vi "Initialize RF Sessions.vi"(0 "RF Subsystem Session Provider in":refnum<class "RF Subsystem Session Provider.lvclass">, 5 "TSM Context":T1, 11 "error in":errorcluster) -> (4 "RF Subsystem Session Provider out":refnum<class "RF Subsystem Session Provider.lvclass">, 15 "error out":errorcluster)   [LabVIEW 2023, in "RFFixtureCharact.RFPM.lvlib" / "RF Subsystem Session Provider.lvclass"]
uses:
  RF Subsystem Session Provider.lvclass
  <vilib>/NI_TestStand_SemiconductorModule/NI_TestStand_Semiconductor_Module.lvlibp/PinMap/General/SemiconductorModuleContext.ctl
  Controls/RFPM Settings.ctl
  Controls/Calibration Check.ctl
  Common/RF Subsystem Session Provider/Utilities/Global Data Id Prefix.vi
  <vilib>/NI_TestStand_SemiconductorModule/NI_TestStand_Semiconductor_Module.lvlibp/PinMap/Site and Global Data/SetGlobalData.vi
  RF Subsystem Session Provider.lvclass/RF Subsystem Session Provider.ctl
  Common/RFCalAndFixtureCharact.Common.lvlib
  <vilib>/NI_TestStand_SemiconductorModule/NI_TestStand_Semiconductor_Module.lvlibp
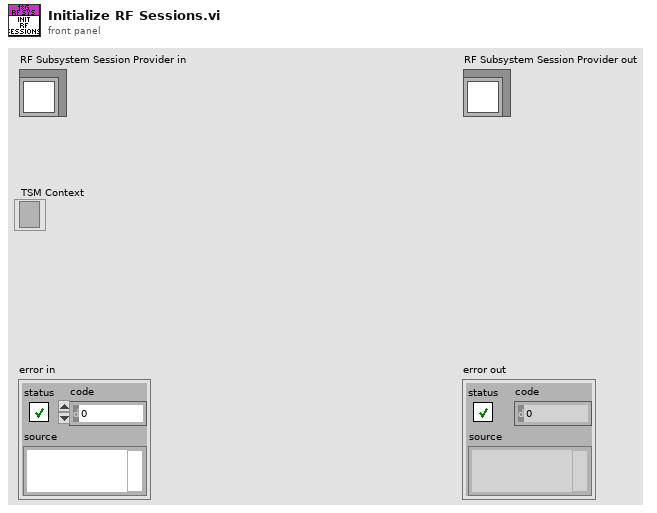
[diagram p1: front panel]
types:
  T1 = typedef "NI_TestStand_Semiconductor_Module.lvlibp/SemiconductorModuleContext.ctl" = refnum<k7>
  T2 = enum16{"OnboardClock", "RefIn", "PXI_Clk", "ClkIn", "RefIn2", "PXI_ClkMaster"}
  T3 = typedef "RFFixtureCharact.RFPM.lvlib/RF Subsystem Session Provider.lvclass/RFPM Settings.ctl" = cluster{"Suppress System Calibration?":bool, "User-Defined Calibration":cluster{"Frequency Interpolation Enabled":bool, "Maximum Frequency Span for Interpolation":dbl, "Source Power Level Coercion Method":i32, "Maximum Source Power Level Coercion":dbl, "Receiver Reference Level Coercion Enabled":bool, "Maximum Receiver Reference Level Coercion":dbl, "Calibration File VST Serial Must Match":bool, "Calibration Interval Check":T4}}
  T4 = typedef "RFFixtureCharact.RFPM.lvlib/RF Subsystem Session Provider.lvclass/Calibration Check.ctl" = cluster{"Check Calibration Interval?":bool, "Temperature Interval (deg C)":dbl, "Calibration Interval (days)":dbl, "Out of Calibration Message":enum16{"Warning", "Error"}}
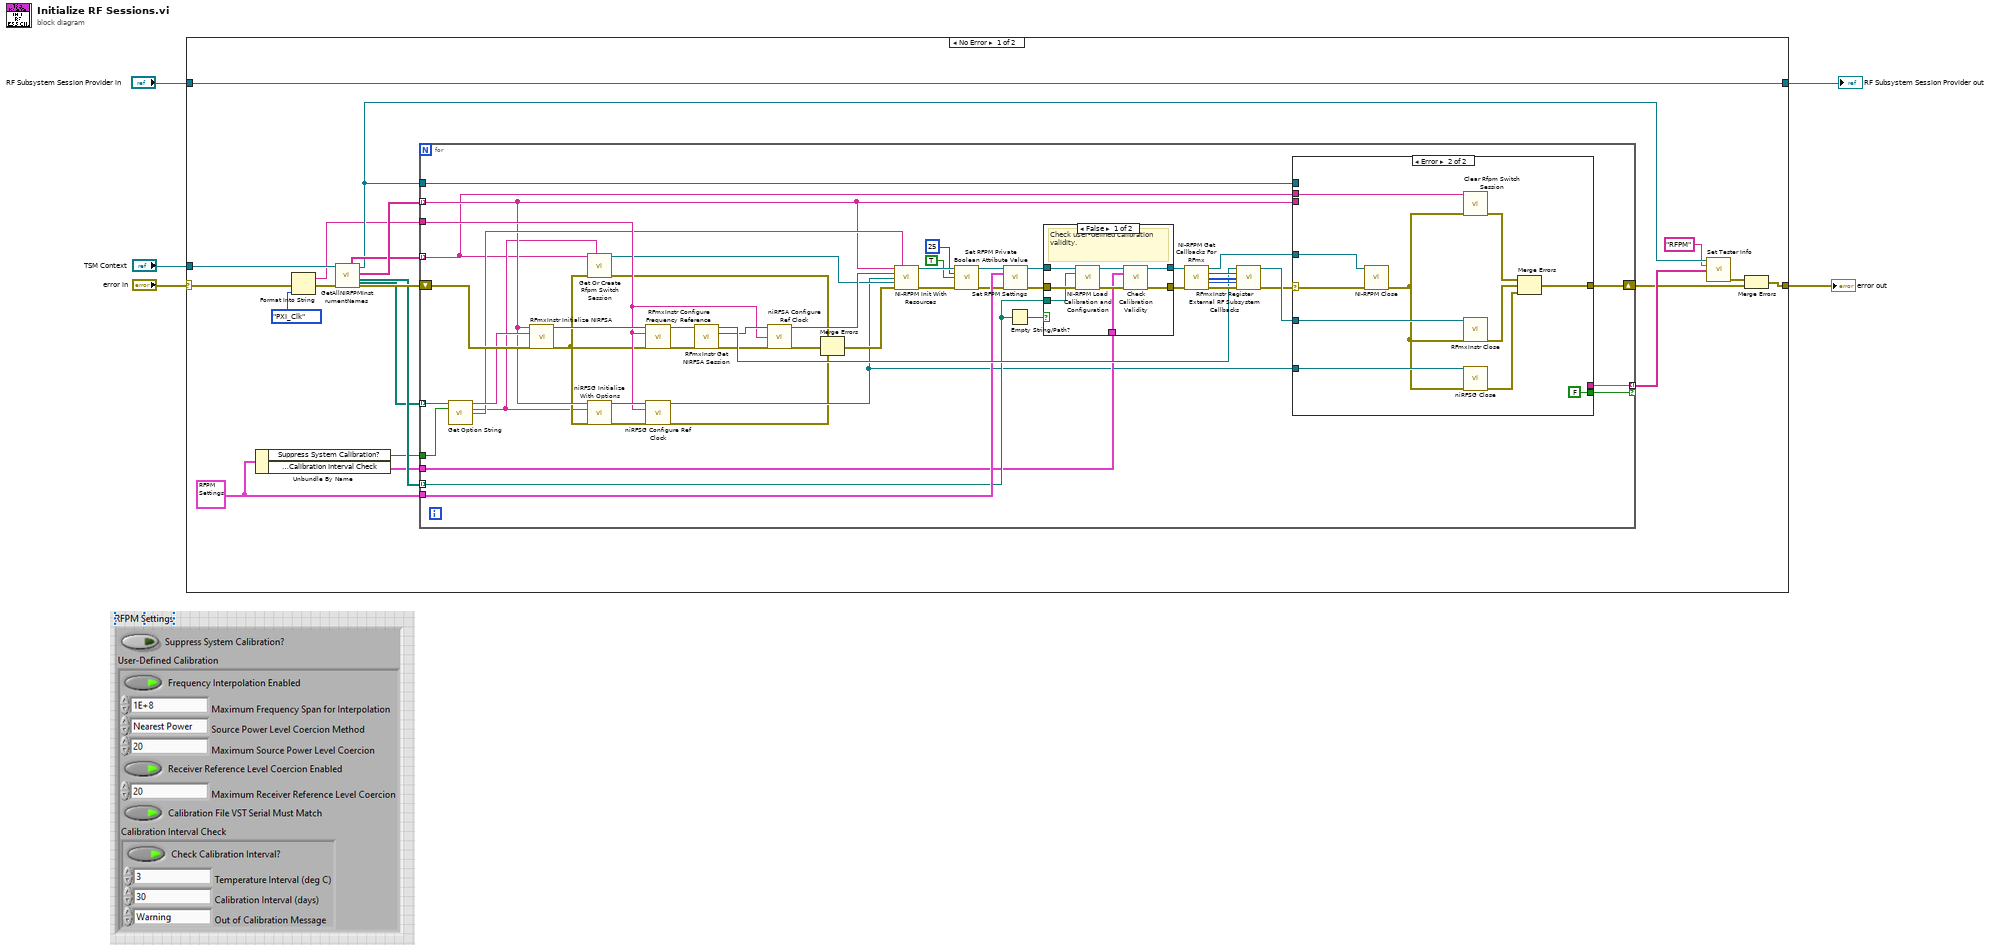
[diagram p0: block diagram]
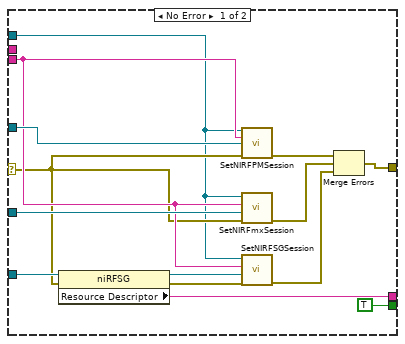
[diagram p3: hidden frame]
diagram:
  n1 = case shown="No Error" "error in" {
    selector: "error in" -> [w15 w112]
    tunnel: [w6 w112] -> w3
    tunnel: "TSM Context" -> [w17 _]
    tunnel: "RF Subsystem Session Provider in" -> [w19 w111]
    tunnel: [w19 w111] -> w1
    frame No Error {
      w18 = T3 {"Suppress System Calibration?"=FALSE, "User-Defined Calibration"={"Frequency Interpolation Enabled"=TRUE, "Maximum Frequency Span for Interpolation"=100000000.0, "Source Power Level Coercion Method"=2, "Maximum Source Power Level Coercion"=20.0, "Receiver Reference Level Coercion Enabled"=TRUE, "Maximum Receiver Reference Level Coercion"=20.0, "Calibration File VST Serial Must Match"=TRUE, "Calibration Interval Check"={"Check Calibration Interval?"=TRUE, "Temperature Interval (deg C)"=3.0, "Calibration Interval (days)"=30.0, "Out of Calibration Message"=enum."Warning"}}} ("RFPM Settings")
      n2 = Unbundle By Name(w18) -> ("Suppress System Calibration?"=w12:bool, "User-Defined Calibration.Calibration Interval Check"=w11:T4)
      n3 = Format Into String(error in=w15, T2."PXI_Clk" ("Reference Clock Source In")) -> (resulting string=w16:string, error out=w14:errorcluster)  [unwired: 2 in]
      n4 = call <vilib>:"GetAllNIRFPMInstrumentNames.vi"("error in (no error)"=w14, "Semiconductor Module Context"=w17) -> ("error out"=w25:errorcluster, "Calibration File Paths"=w23:path[], "Instrument Names"=w24:string[], "Semiconductor Module Context out"=w20:T1, "IVI Switch Names"=w21:string[], "FPGA File Paths"=w22:path[])  [unwired: 4 in]
      n5 = for {
        tunnel: w24 -> [w51] mode=indexing
        tunnel: w23 -> [w38] mode=indexing
        tunnel: w20 -> [w74]
        shift-right: [w73] -> w7
        shift-left: w25 -> [w60]
        tunnel: w22 -> [w55] mode=indexing
        tunnel: w21 -> [w35] mode=indexing
        tunnel: w16 -> [w59]
        tunnel: w18 -> [w44]
        tunnel: w12 -> [w54]
        tunnel: [w50] -> w9 mode=indexing if=w49
        tunnel: w11 -> [w37]
        n6 = call "Get Option String.vi"("FPGA File Path"=w55, "Suppress System Calibration?"=w54) -> ("RFmx Option String"=w53:string, "FPGA Option String"=w36:string, "RFPM Option String"=w52:string)  [unwired: 11 in]
        n7 = call <vilib>:"RFmxInstr Initialize NIRFSA.vi"("Resource Name"=w51, "Option String"=w53, "error in (no error)"=w60) -> ("Instrument Handle Out"=w64:refnum<k21>, "error out"=w46:errorcluster)  [unwired: 10 in, 1 out]
        n8 = call "Get Or Create Rfpm Switch Session.vi"("logical name (\"SampleSwitch\")"=w35, "option string (\"Simulate=0,RangeCheck=1,QueryInstrStatus=0,Cache=1\")"=w36, "error in (no error)"=w46) -> ("Ivi Switch Session out"=w48:refnum<k15>, "error out"=w47:errorcluster)  [unwired: 11 in]
        n9 = call <instrlib>:"niRFSG Initialize With Options.vi"("resource name"=w51, "option string"=w36, "error in"=w46) -> ("instrument handle"=w72:refnum<k15>, "error out"=w75:errorcluster)  [unwired: 11 in]
        n10 = call <vilib>:"RFmxInstr Configure Frequency Reference.vi"("Instrument Handle In"=w64, "Frequency Reference Source"=w59, "error in (no error)"=w46) -> ("Instrument Handle Out"=w28:refnum<k21>, "error out"=w29:errorcluster)  [unwired: 11 in]
        n11 = call <instrlib>:"niRFSG Configure Ref Clock.vi"("instrument handle"=w72, "ref clock source"=w59, "error in"=w75) -> ("instrument handle out"=w27:refnum<k15>, "error out"=w26:errorcluster)  [unwired: 11 in]
        n12 = call <vilib>:"RFmxInstr Get NIRFSA Session.vi"("Instrument Handle In"=w28, "error in (no error)"=w29) -> ("Instrument Handle Out"=w65:refnum<k21>, "NI RFSA Session"=w63:refnum<k15>, "error out"=w61:errorcluster)  [unwired: 11 in]
        n13 = call <instrlib>:"niRFSA Configure Ref Clock.vi"("instrument handle"=w63, "clock source"=w59, "error in"=w61) -> ("instrument handle out"=w58:refnum<k15>, "error out"=w62:errorcluster)  [unwired: 11 in]
        n14 = Merge Errors(w47, w62, w26) -> (w57:errorcluster)
        n15 = call <instrlib>:"NI-RFPM Init With Resources.vi"("resource name"=w51, "option string"=w52, "RFSA handle"=w58, "RFSG handle"=w27, "Switch handle"=w48, "error in"=w57) -> ("instrument handle out"=w33:refnum<k15>, "error out"=w45:errorcluster)  [unwired: 8 in]
        n16 = call "Set RFPM Private Boolean Attribute Value.vi"("reference"=w33, "Attribute"=25, "value"=TRUE, "error in"=w45) -> ("reference out"=w32:refnum<k15>, "error out"=w34:errorcluster)  [unwired: 10 in]
        n17 = call "Set RFPM Settings.vi"("RFPM Handle In"=w32, "RFPM Settings"=w44, "error in"=w34) -> ("RFPM Handle Out"=w43:refnum<k15>, "error out"=w42:errorcluster)  [unwired: 11 in]
        n18 = Empty String/Path?(string/path=w38) -> (empty?=w39:bool)
        n19 = case shown="False" w39 {
          tunnel: w43 -> [w83 w85]
          tunnel: w42 -> [w82 w84]
          tunnel: [w79 w85] -> w41
          tunnel: [w78 w84] -> w40
          tunnel: w38 -> [w77 _]
          tunnel: w37 -> [w76 _]
          frame False {
            # "Check user-defined calibration validity."
            n20 = call <instrlib>:"NI-RFPM Load Calibration and Configuration.vi"("NI-5530 handle in"=w83, "Calibration Storage File Path"=w77, "error in"=w82) -> ("instrument handle out"=w81:refnum<k15>, "error out"=w80:errorcluster)  [unwired: 11 in]
            n21 = call "Check Calibration Validity.vi"("RFPM Handle In"=w81, "Calibration Interval Check"=w76, "error in"=w80) -> ("RFPM Handle Out"=w79:refnum<k15>, "error out"=w78:errorcluster)  [unwired: 11 in]
          }
          frame True {
          }
        }
        n22 = call <instrlib>:"NI-RFPM Get Callbacks For RFmx.vi"("instrument handle"=w41, "error in"=w40) -> ("instrument handle out"=w70:refnum<k15>, "Context"=w69:u64, "Callbacks For RFmx"=w68:u64[], "Callback Version"=w67:i32, "error out"=w71:errorcluster)  [unwired: 9 in]
        n23 = call <vilib>:"RFmxInstr Register External RF Subsystem Callbacks.vi"("Instrument Handle In"=w65, "External RF Subsystem Context"=w69, "Callbacks"=w68, "Callback Version"=w67, "error in (no error)"=w71) -> ("Instrument Handle Out"=w66:refnum<k21>, "error out"=w56:errorcluster)  [unwired: 9 in]
        n24 = case shown="Error" w56 {
          selector: w56 -> [w89 w102]
          tunnel: [w99 w110] -> w73
          tunnel: w70 -> [w98 w108]
          tunnel: w35 -> [_ w109]
          tunnel: w74 -> [w86 _]
          tunnel: w66 -> [w96 w106]
          tunnel: w27 -> [w97 w107]
          tunnel: w51 -> [w92 _]
          tunnel: [w88 _] -> w50
          tunnel: [TRUE FALSE] -> w49
          frame No Error {
            n25 = property class="niRFSG"(reference=w97, error in=w89) -> (reference out=w91:refnum<k15>, error out=w90:errorcluster, "Resource Descriptor"=w88:string)
            n26 = call <vilib>:"SetNIRFPMSession.vi"("Semiconductor Module Context"=w86, "Instrument Name"=w92, "NI-RFPM Session"=w98, "error in (no error)"=w89) -> ("error out"=w94:errorcluster)  [unwired: 10 in, 1 out]
            n27 = call <vilib>:"SetNIRFmxSession.vi"("error in (no error)"=w89, "NI-RFmx Session"=w96, "Instrument Name"=w92, "Semiconductor Module Context"=w86) -> ("error out"=w95:errorcluster)  [unwired: 6 in, 1 out]
            n28 = call <vilib>:"SetNIRFSGSession.vi"("error in (no error)"=w90, "NI-RFSG Session"=w91, "Instrument Name"=w92, "Semiconductor Module Context"=w86) -> ("error out"=w93:errorcluster)  [unwired: 6 in, 1 out]
            n29 = Merge Errors(w94, w95, w93) -> (w99:errorcluster)
          }
          frame Error {
            n30 = call <instrlib>:"NI-RFPM Close.vi"("NI-5530 handle in"=w108, "error in"=w102) -> ("error out"=w101:errorcluster)  [unwired: 13 in]
            n31 = call "Clear Rfpm Switch Session.vi"("Logical Name"=w109, "error in (no error)"=w101) -> ("error out"=w100:errorcluster)  [unwired: 13 in]
            n32 = call <vilib>:"RFmxInstr Close.vi"("Instrument Handle In"=w106, "error in (no error)"=w101) -> ("error out"=w105:errorcluster)  [unwired: 13 in]
            n33 = call <instrlib>:"niRFSG Close.vi"("instrument handle"=w107, "error in"=w101) -> ("error out"=w104:errorcluster)  [unwired: 13 in]
            n34 = Merge Errors(w100, w105, w104) -> (w110:errorcluster)
          }
        }
      }
      n35 = call "Set Tester Info.vi"("TSM Context In"=w20, "Tester Type"="RFPM", "Resource Descriptors"=w9) -> ("error out"=w8:errorcluster)  [unwired: 11 in, 1 out]
      n36 = Merge Errors(w8, w7) -> (w6:errorcluster)
    }
    frame Error {
    }
  }
  "error out" <- w3
  "RF Subsystem Session Provider out" <- w1
